vi "Process_SetDataUnlock.vi"(0 "ref in":T2, 1 "Lock ref in":T1, 2 "Data in":T3, 3 "error in":errorcluster) -> (6 "ref out":T2, 9 "error out":errorcluster)   [LabVIEW 2015]
uses:
  Control/Process_Data.ctl
  Control/Process_Mode.ctl
  Control/Process_Function.ctl
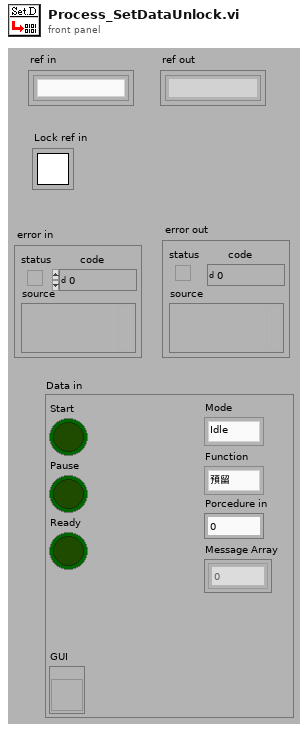
[diagram p1: front panel]
types:
  T1 = typedef "Semaphore RefNum" = refnum<k1>
  T2 = typedef "Error站_ref.ctl" = refnum<k1>
  T3 = typedef "Process_Data.ctl" = cluster{"GUI":refnum<vi>, "Ready":bool, "Mode":T4, "Function":T5, "Porcedure in":u8, "Message Array":i32[], "Start":bool, "Pause":bool}
  T4 = typedef "Process_Mode.ctl" = enum8{"Idle", "Run", "Pause", "Err"}
  T5 = typedef "Process_Function.ctl" = enum8{"預留"}
  T6 = enum16{"OpenReference", "CloseReference", "Get Data", "Set Data", "Set Flag"}
  T7 = typedef "Process_ref.ctl" = refnum<k1>
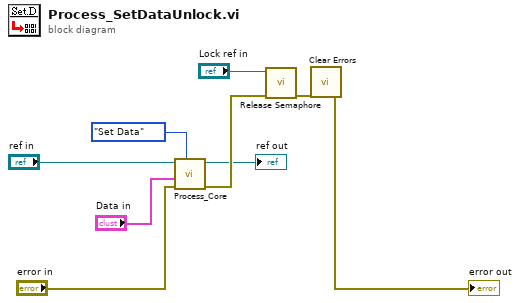
[diagram p0: block diagram]
diagram:
  n1 = call "Process_Core.vi"("Function"=T6."Set Data", "error in"="error in", "Data in"="Data in", "ref in"="ref in") -> ("error out"=w9:errorcluster, "ref out"=→"ref out":T7)  [unwired: 4 in, 2 out]
  n2 = call <vilib>:"Release Semaphore.vi"("error in (no error)"=w9, "semaphore"="Lock ref in") -> ("error out"=w5:errorcluster)  [unwired: 4 in, 1 out]
  n3 = call <vilib>:"Clear Errors.vi"("error in (no error)"=w5) -> ("error out"=→"error out":errorcluster)  [unwired: 5 in, 1 out]
